vi "Count Data Valids (U32).vi"(2 "Reset?":bool, 7 "Data Valid":bool) -> (8 "Counter":u32)   [LabVIEW 2012]
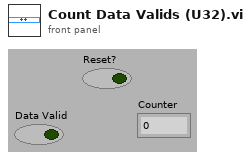
[diagram p1: front panel]
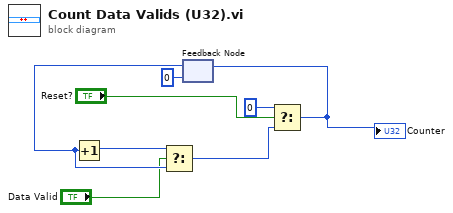
[diagram p0: block diagram]
diagram:
  n1 = feedback #1(u32 0 ("t")) -> (w3:u32)
  n2 = Increment(x=w3) -> (x+1=w4:u32)
  n3 = Select(t=w4, s="Data Valid", f=w3) -> (s? t:f=w1:u32)
  n4 = Select(t=u32 0, s="Reset?", f=w1) -> (s? t:f=w8:u32)
  "Counter" <- w8
  n5 = feedback-in #1(w8) -> ()
